vi "Search for Sequence.vi"(4 "Tower Heights":map{i32, u64}(c390), 5 "Settled Rocks":i32[](array[numeric]), 6 "Sequence Found ? in":bool, 9 "Sequence Analysis in":T1) -> (0 "Sequence Found ? out":bool, 3 "Sequence Analysis out":T1)   [LabVIEW 2020, in "AoC 2022.lvlib"]
uses:
  AoC 2022.lvlib
  Sequence Analysis.ctl
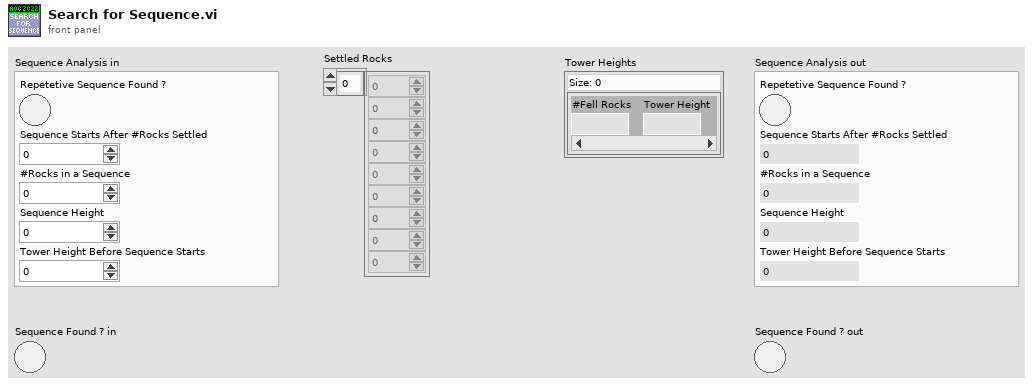
[diagram p1: front panel]
types:
  T1 = typedef "AoC 2022.lvlib/Sequence Analysis.ctl" = cluster{"Repetetive Sequence Found ?":bool, "Sequence Starts After #Rocks Settled":i32, "#Rocks in a Sequence":i32, "Sequence Height":u64, "Tower Height Before Sequence Starts":u64}
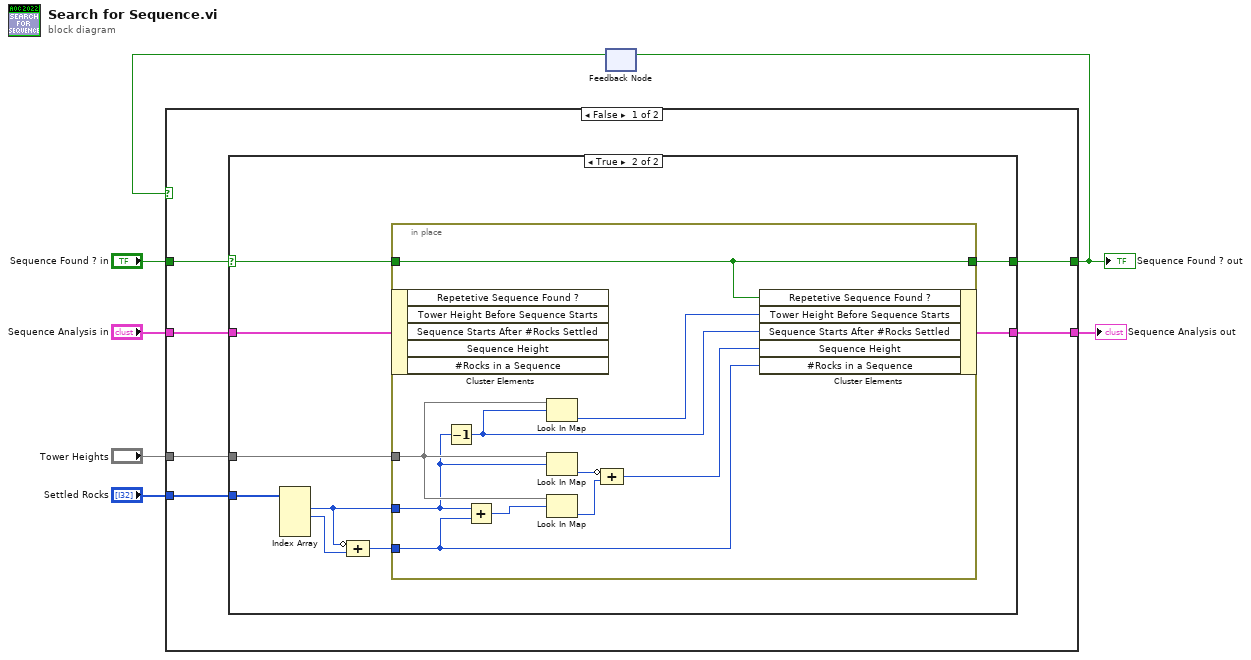
[diagram p0: block diagram]
diagram:
  n1 = feedback #1() -> (w1:bool)  [unwired: 1 in]
  n2 = case shown="False" w1 {
    tunnel: "Settled Rocks" -> [w9 _]
    tunnel: "Sequence Analysis in" -> [w13 w36]
    tunnel: [w12 w36] -> w5
    tunnel: [w11 w35] -> w2
    tunnel: "Tower Heights" -> [w10 _]
    tunnel: "Sequence Found ? in" -> [w8 w35]
    frame False {
      n3 = case shown="True" w8 {
        selector: w8 -> [w15 w16]
        tunnel: w13 -> [w14 w24]
        tunnel: [w14 w23] -> w12
        tunnel: [w15 w22] -> w11
        tunnel: w10 -> [_ w21]
        tunnel: w9 -> [_ w20]
        frame False {
        }
        frame True {
          n4 = Index Array(array=w20) -> (element #1=w18:i32, element #2=w19:i32)  [unwired: 4 in, 2 out]
          n5 = Compound Arithmetic op=ADD(invert w18, w19) -> (w17:i32)
          n6 = in-place {
            in-place-border: [w25] -> w22
            in-place-border: w17 -> [w27]
            in-place-border: w21 -> [w31]
            in-place-border: w18 -> [w30]
            in-place-border: w16 -> [w25]
            n7 = in-place-cluster #2(w24) -> ()  [unwired: 5 out]
            n8 = Decrement(x=w30) -> (x-1=w28:i32)
            n9 = Add(x=w30, y=w27) -> (x+y=w29:i32)
            n10 = Look In Map(map=w31, key=w28) -> (value=w26:u64)  [unwired: 1 in, 1 out]
            n11 = Look In Map(map=w31, key=w30) -> (value=w34:u64)  [unwired: 1 in, 1 out]
            n12 = Look In Map(map=w31, key=w29) -> (value=w33:u64)  [unwired: 1 in, 1 out]
            n13 = Compound Arithmetic op=ADD(invert w34, w33) -> (w32:u64)
            n14 = in-place-cluster #2("Repetetive Sequence Found ?"=w25, "Tower Height Before Sequence Starts"=w26, "Sequence Starts After #Rocks Settled"=w28, "Sequence Height"=w32, "#Rocks in a Sequence"=w27) -> (w23:T1)
          }
        }
      }
    }
    frame True {
    }
  }
  "Sequence Found ? out" <- w2
  "Sequence Analysis out" <- w5
  n15 = feedback-in #1(w2) -> ()
